vi "Chirp Demo-1.vi"() -> ()   [LabVIEW 2015]
uses:
  Utility VIs/Math VIs/FFT x(t) to dB,Degrees (1D).vi
panel:
  out "Data.WF":dbl[][](array[numeric])
  out "Elapsed time (ms/chirp)":dbl=0.169
  in  "Compensate":bool
  out "Magnitude graph":cluster{"Array":dbl[], "Array":dbl[]}(graph)={"Array"=[0.0, 0.5, 1.0, 1.5, 2.0, 2.5, 3.0, 3.5, 4.0, 4.5, 5.0, 5.5, 6.0, 6.5, 7.0, 7.5, 8.0, 8.5, 9.0, 9.5, 10.0, 10.5, 11.0, 11.5, 12.0, 12.5, 13.0, 13.5, 14.0, 14.5, 15.0, 15.5, 16.0, 16.5, 17.0, 17.5, 18.0, 18.5, 19.0, 19.5, 20.0, 20.5, 21.0, 21.5, 22.0, 22.5, 23.0, 23.5, 24.0, 24.5, 25.0, 25.5, 26.0, 26.5, 27.0, 27.5, 28.0, 28.5, 29.0, 29.5, 30.0, 30.5, 31.0, 31.5, 32.0, 32.5, 33.0, 33.5, 34.0, 34.5, 35.0, 35.5, 36.0, 36.5, 37.0, 37.5, 38.0, 38.5, 39.0, 39.5, 40.0, 40.5, 41.0, 41.5, 42.0, 42.5, 43.0, 43.5, 44.0, 44.5, 45.0, 45.5, 46.0, 46.5, 47.0, 47.5, 48.0, 48.5, 49.0, 49.5, 50.0, 50.5, 51.0, 51.5, 52.0, 52.5, 53.0, 53.5, 54.0, 54.5, 55.0, 55.5, 56.0, 56.5, 57.0, 57.5, 58.0, 58.5, 59.0, 59.5, 60.0, 60.5, 61.0, 61.5, 62.0, 62.5, 63.0, 63.5, 64.0, 64.5, 65.0, 65.5, 66.0, 66.5, 67.0, 67.5, 68.0, 68.5, 69.0, 69.5, 70.0, 70.5, 71.0, 71.5, 72.0, 72.5, 73.0, 73.5, 74.0, 74.5, 75.0, 75.5, 76.0, 76.5, 77.0, 77.5, 78.0, 78.5, 79.0, 79.5, 80.0, 80.5, 81.0, 81.5, 82.0, 82.5, 83.0, 83.5, 84.0, 84.5, 85.0, 85.5, 86.0, 86.5, 87.0, 87.5, 88.0, 88.5, 89.0, 89.5, 90.0, 90.5, 91.0, 91.5, 92.0, 92.5, 93.0, 93.5, 94.0, 94.5, 95.0, 95.5, 96.0, 96.5, 97.0, 97.5, 98.0, 98.5, 99.0, 99.5], "Array"=[-20.36394181934157, -23.007216204012373, -31.418402002400462, -53.43578131991167, -40.8136242465494, -39.42735683064596, -44.505148407086104, -32.39813684405413, -24.159544929918717, -22.68134967914014, -26.499784232581757, -49.67783033258621, -32.2052191082686, -51.634738674411565, -26.711578041233256, -28.614808505293293, -28.28225482008967, -26.872390354366598, -29.07672981153116, -27.083867467170997, -23.675395212630164, -25.15425132427353, -61.51620440248326, -33.50112317092914, -45.42769977720599, -31.419246348241174, -39.2682099993328, -33.70315980719094, -32.62888074080665, -26.706378589678586, -24.64711828051657, -36.33896465774261, -34.509174932360224, -35.05324004816531, -43.14378431280592, -62.24651581738131, -38.155558870061554, -37.345933071293146, -27.514185458741164, -32.17763642678305, -22.206346063587908, -25.311338819931354, -27.02662562007994, -24.496856107361346, -26.993865625667425, -46.57555656335142, -32.00950126411297, -41.203693083398996, -51.77571051875478, -30.70109339292971, -22.0467659143819, -24.054893657186195, -34.623970763372014, -36.464874852537335, -26.58467623001342, -30.678558440606018, -39.64424340237133, -28.302680006372185, -26.574423737895355, -32.93745936323169, -35.2687296616985, -29.457695476121405, -32.99905004866836, -37.02911649267071, -31.366198628838546, -37.705983062922506, -34.13614785816253, -33.741854251786606, -37.01864471864471, -27.55923346348268, -26.05912873474496, -41.493053280167885, -23.245362240408937, -27.519458073098004, -31.497964196178103, -24.939615396835315, -24.387887947551885, -38.886908114842825, -30.540613911342042, -38.69828950114367, -43.41703617377021, -27.384033807485437, -32.55675114967582, -39.44683315946287, -38.53811339243861, -55.11962338317812, -42.73334249000907, -34.53597280249117, -29.191586481586214, -30.366227831521385, -41.85510754680522, -56.982457663469106, -42.24168747593396, -35.974247329657, -33.66734884051944, -35.30220244186906, -32.09534523815597, -26.2751841805029, -34.89656678531133, -41.9407733950674, -38.881134206252156, -40.3974086976455, -35.56028925953045, -41.71707820522313, -34.18468007661665, -30.007477020363204, -59.32872762809708, -55.74835971630912, -33.285570630788534, -45.99965994385083, -28.196144966960045, -28.895203634521707, -34.629829452425994, -33.15500302376064, -37.19071906405268, -55.16841487859309, -30.05351082894848, -26.483876200637884, -45.74381635211598, -32.65354287040351, -34.57298379405399, -45.3981061572107, -36.79718243178327, -29.02665699163164, -31.679732317092572, -34.96855029056365, -34.43444410534666, -56.80334086722729, -46.43551827714993, -46.17765256883213, -43.724732396023796, -52.686369953594465, -36.901054491695, -28.511298209229707, -29.928868152110336, -43.80246715440058, -46.8833561276006, -67.40798262010874, -31.86817760204265, -32.903068661686476, -47.37216389157285, -41.190692210331264, -35.14335583047213, -43.939511005729955, -34.48683485417986, -42.985124405214776, -34.36475319589025, -34.039079011391394, -38.877149767228, -66.93827647848737, -39.586945407216376, -47.475865022837375, -30.719504201064925, -41.68538762080289, -37.026871725631366, -37.960891744204034, -25.288114548098587, -30.726414767121888, -33.2564879998464, -43.36489389299061, -33.74154522789504, -29.6837389680518, -29.254222110517112, -55.26384587618338, -45.42333366437664, -32.25318219703378, -31.187671789275292, -48.271365047159584, -33.2999121991835, -51.82455459163589, -43.76730876147051, -37.400147046577175, -38.66872438484014, -38.31484115087673, -31.839671836215192, -30.087088073072984, -34.70316958689242, -45.70416173145314, -38.84711654227978, -29.726760894405487, -30.18586090581803, -34.50598024287888, -29.090565251988583, -32.296337502665864, -36.54110786709963, -46.91632210527506, -32.64339816950588, -35.168573317531376, -28.777992098118336, -25.57751731903061, -31.610741535687232, -40.91295864063557, -34.592716546891246, -32.38415090421482, -48.95920522803404, -43.73578166751365, -33.78531553386493, -35.10115333441517, -42.367281574644636, -25.740182862511425]}
  out "Signal graph":cluster{"Array":dbl[], "Array":dbl[]}(graph)
  in  "Duration (ms)":dbl=2.0
  in  "Fmax (kHz)":dbl=64.0
  in  "Fmin (kHz)":dbl=4.0
  in  "Fs (Hz)":dbl=200000.0
  out "Calibration":cluster{"Frequency (Hz)":dbl[], "Mag":dbl[]}(graph)
  in  "Calibration file":path=path "C:/Data/XYZ DATA/XYZ999/RightPrimary.calib"
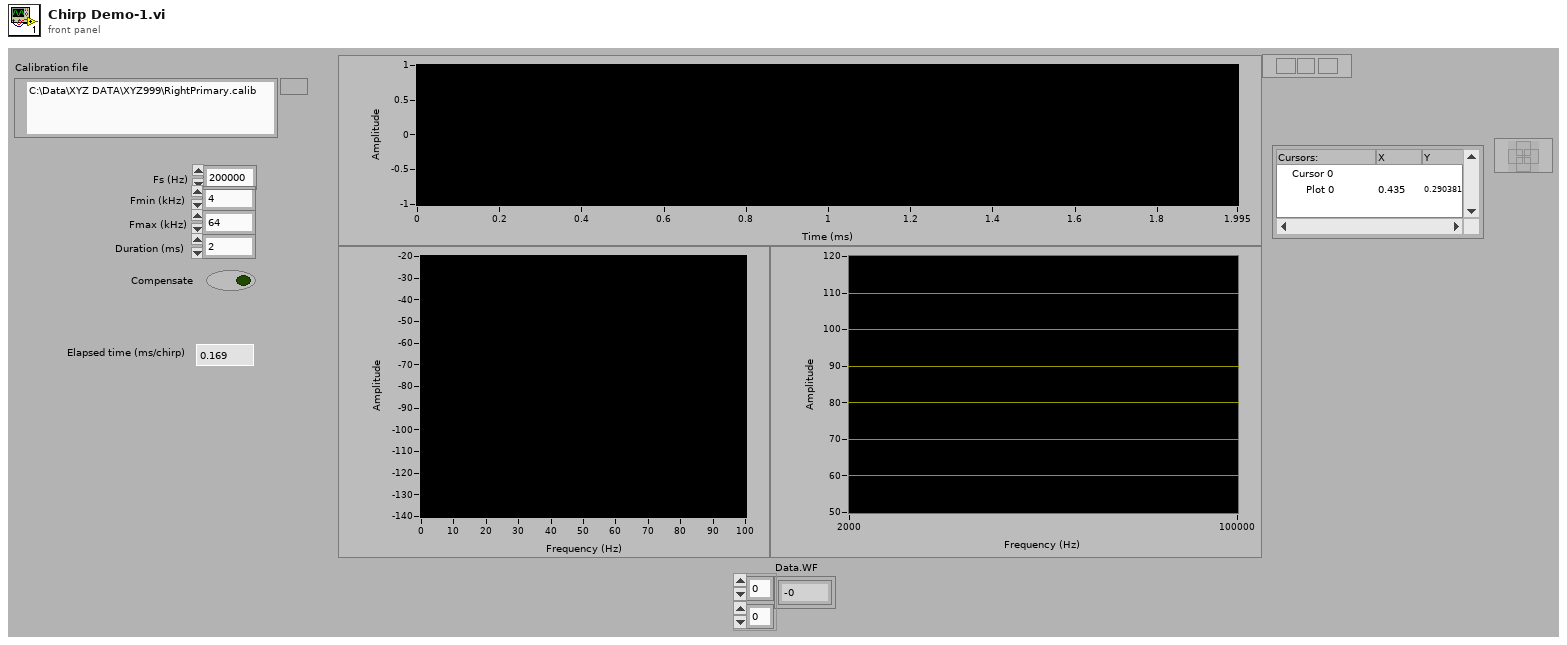
[diagram p1: front panel]
types:
  T1 = cluster{"Frequency (Hz)":dbl[], "Mag":dbl[], "Phase":dbl[]}
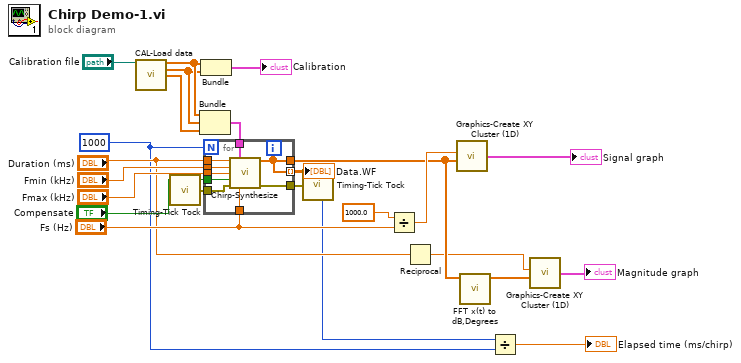
[diagram p0: block diagram]
diagram:
  w2 = 1000
  n1 = call "CAL-Load data.vi"("user path"="Calibration file") -> ("Frequency (Hz)"=w10:dbl[], "Mag"=w9:dbl[], "Phase"=w8:dbl[])  [unwired: 7 in, 5 out]
  n2 = call "Timing-Tick Tock.vi"() -> ("error out"=w6:errorcluster)  [unwired: 6 in, 1 out]
  n3 = Bundle("Frequency (Hz)"=w10, "Mag"=w9, "Phase"=w8) -> (w7:T1)  [unwired: 1 in]
  n4 = Bundle("Frequency (Hz)"=w10, "Mag"=w9) -> (→"Calibration":cluster{"Frequency (Hz)":dbl[], "Mag":dbl[]})  [unwired: 1 in]
  n5 = for {
    N: w2 -> [_]
    tunnel: "Fmin (kHz)" -> [w33]
    tunnel: "Fmax (kHz)" -> [w32]
    tunnel: "Compensate" -> [w31]
    tunnel: "Fs (Hz)" -> [w30]
    tunnel: [w25] -> w17
    tunnel: "Duration (ms)" -> [w29]
    tunnel: w7 -> [w28]
    tunnel: w6 -> [w27]
    tunnel: [w26] -> w5
    tunnel: [w25] -> w1 mode=indexing
    n6 = call "Chirp-Synthesize.vi"("Duration (ms)"=w29, "Cal"=w28, "Fmin (kHz)"=w33, "Fmax (kHz)"=w32, "Compensate"=w31, "error in (no error)"=w27, "Sampling rate (Hz)"=w30) -> ("Data.WF"=w25:dbl[], "error out"=w26:errorcluster)  [unwired: 7 in]
  }
  "Data.WF" <- w1
  n7 = call "Timing-Tick Tock.vi"("error in (no error)"=w5) -> ("Elapsed time (ms)"=w4:u32)  [unwired: 5 in, 1 out]
  n8 = Divide(x=1000.0, y="Fs (Hz)") -> (x/y=w19:dbl)
  n9 = Reciprocal(x="Duration (ms)") -> (1/x=w14:dbl)
  n10 = call "Graphics-Create XY Cluster (1D).vi"("Array"=w17, "dx"=w19) -> ("XY cluster"=→"Signal graph":cluster{"Array":dbl[], "Array":dbl[]})  [unwired: 2 in]
  n11 = call-poly "FFT x(t) to dB,Degrees.vi"("X"=w17) -> ("+Freq. Mag of FFT (dB rms)"=w15:dbl[])  [unwired: 8 in, 2 out]
  n12 = Divide(x=w4, y=w2) -> (x/y=→"Elapsed time (ms/chirp)":dbl)
  n13 = call "Graphics-Create XY Cluster (1D).vi"("Array"=w15, "dx"=w14) -> ("XY cluster"=→"Magnitude graph":cluster{"Array":dbl[], "Array":dbl[]})  [unwired: 2 in]
